vi "Run Icon Editor from Source Selector.vi"(11 "Inputs":string[](array[string])=["", ""]) -> (2 "Output/Failure":string, 3 "CLI Process Return Code":i32)   [LabVIEW 2021]
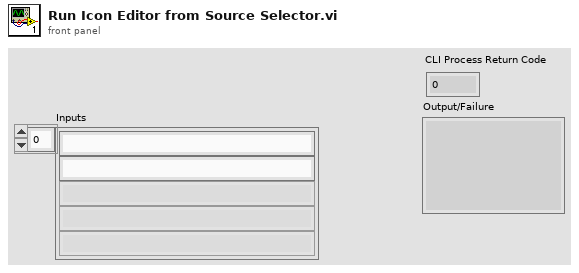
[diagram p1: front panel]
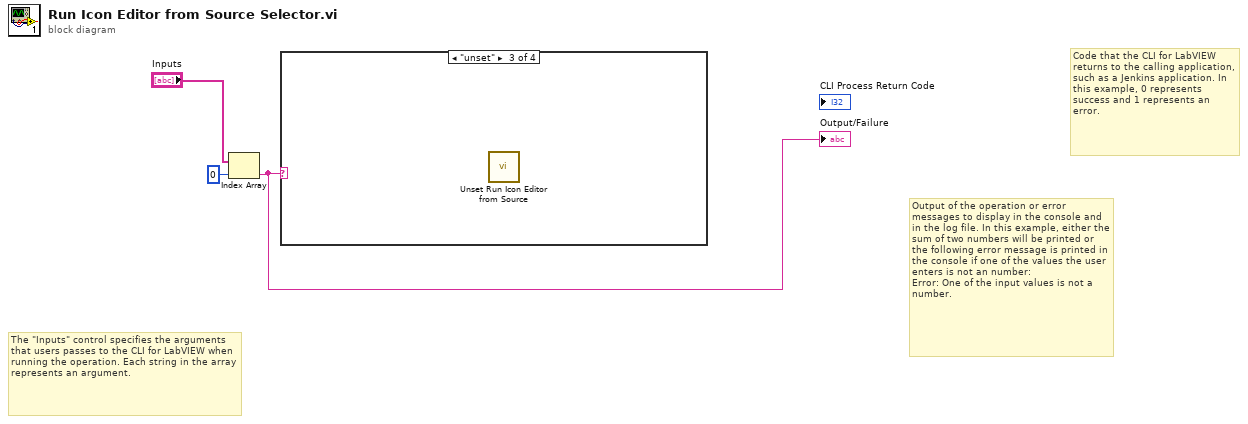
[diagram p0: block diagram]
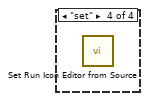
[diagram p4: hidden frame]
diagram:
  # "Output of the operation or error messages to display in the console and in the log file. In this example, either the sum of two numbers will be printed or the following error message is printed in the console if one of the values the user enters is not an number:\nError: One of the input values is not a number."
  # "Code that the CLI for LabVIEW returns to the calling application, such as a Jenkins application. In this example, 0 represents success and 1 represents an error."
  # "The \"Inputs\" control specifies the arguments that users passes to the CLI for LabVIEW when running the operation. Each string in the array represents an argument."
  n1 = Index Array(array="Inputs", index=0) -> (element=w1:string)
  "Output/Failure" <- w1
  n2 = case shown="\"unset\"" w1 {
    frame Default {
    }
    frame "skip" {
    }
    frame "unset" {
      n3 = call "Unset Run Icon Editor from Source.vi"() -> ()  [unwired: 12 in]
    }
    frame "set" {
      n4 = call "Set Run Icon Editor from Source.vi"() -> ()  [unwired: 12 in]
    }
  }
